vi "ForLoopExample.vi"() -> ()   [LabVIEW 2020]
panel:
  out "Numer iteracji":i32
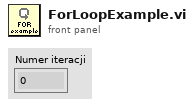
[diagram p1: front panel]
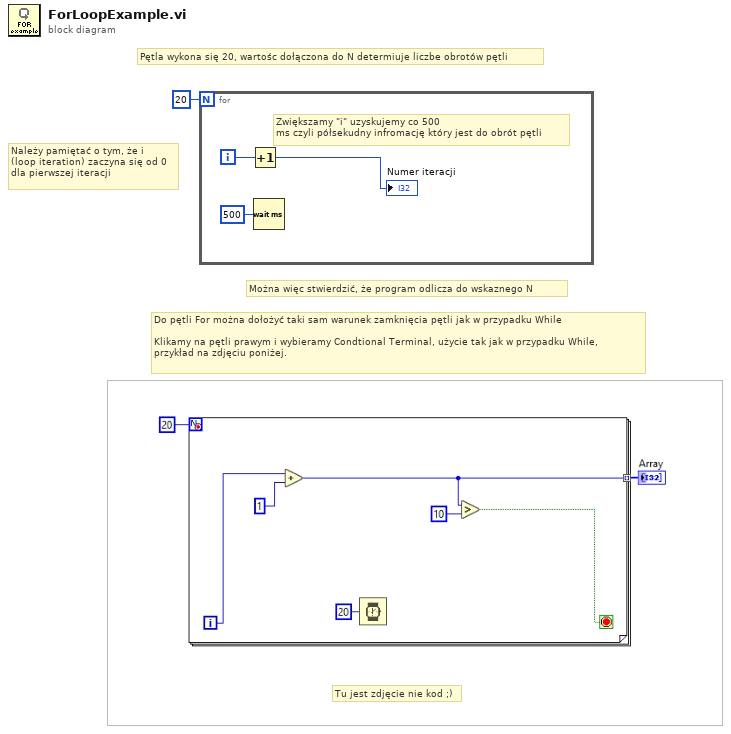
[diagram p0: block diagram]
diagram:
  # "Tu jest zdjęcie nie kod ;)"
  # "Do pętli For można dołożyć taki sam warunek zamknięcia pętli jak w przypadku While\n\nKlikamy na pętli prawym i wybieramy Condtional Terminal, użycie tak jak w przypadku While,\nprzykład na zdjęciu poniżej."
  # "Można więc stwierdzić, że program odlicza do wskaznego N"
  # "Należy pamiętać o tym, że i \n(loop iteration) zaczyna się od 0\ndla pierwszej iteracji"
  # "Pętla wykona się 20, wartośc dołączona do N determiuje liczbe obrotów pętli"
  n1 = for {
    N: 20 -> [_]
    i -> [w4]
    # "Zwiększamy \"i\" uzyskujemy co 500\nms czyli półsekudny infromację który jest do obrót pętli"
    n2 = Increment(x=w4) -> (x+1=→"Numer iteracji":i32)
    n3 = Wait (ms)(milliseconds to wait=u32 500) -> ()  [unwired: 1 out]
  }
